vi "Format Output.vi"(8 "error in (no error)":errorcluster, 10 "Input":string, 11 "Fluke Calibrator in":refnum<class "Fluke Calibrator.lvclass">) -> (0 "error out":errorcluster, 2 "Output":bool, 3 "Fluke Calibrator out":refnum<class "Fluke Calibrator.lvclass">)   [LabVIEW 2012, in "Fluke Calibrator.lvclass"]
uses:
  Fluke Calibrator.lvclass
  Fluke Calibrator.lvclass/Fluke Calibrator.ctl
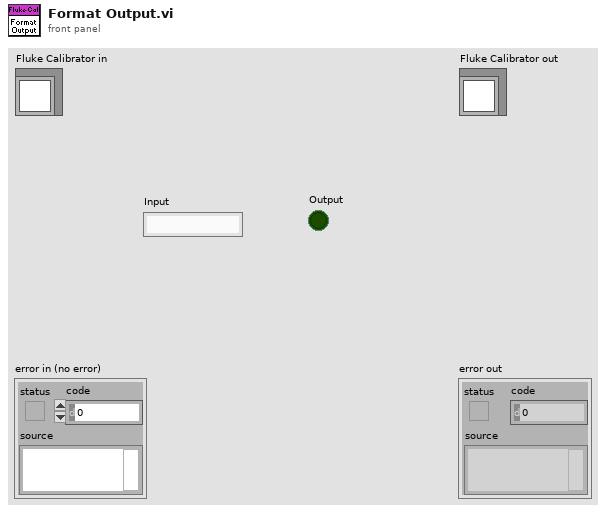
[diagram p1: front panel]
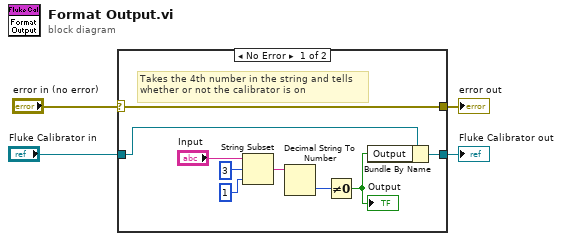
[diagram p0: block diagram]
diagram:
  n1 = case shown="No Error" "error in (no error)" {
    selector: "error in (no error)" -> [w13 w15]
    tunnel: [w13 w15] -> w3
    tunnel: [w6 w14] -> w1
    tunnel: "Fluke Calibrator in" -> [w7 w14]
    frame No Error {
      # "Takes the 4th number in the string and tells whether or not the calibrator is on"
      n2 = String Subset(string="Input", offset (0)=3, length (rest)=1 ("length (rest)")) -> (substring=w10:string)
      n3 = Decimal String To Number(string=w10) -> (number=w9:i32)  [unwired: 2 in, 1 out]
      n4 = Not Equal To 0?(x=w9) -> (x != 0?=w5:bool)
      "Output" <- w5
      n5 = Bundle By Name(cluster=w7, "Output"=w5) -> (w6:refnum<class "Fluke Calibrator.lvclass">)
    }
    frame Error {
    }
  }
  "error out" <- w3
  "Fluke Calibrator out" <- w1
